vi "FieldScouting.vi"() -> ()   [LabVIEW 2015]
uses:
  <vilib>/Utility/sysdir.llb/System Directory Type.ctl
panel:
  in  "Comments":string
  in  "Low Goals Auto":dbl format="%#_4g"
  in  "High Goals Auto":dbl format="%#_4g"
  in  "?":bool
  in  "Rating":dbl=1.0 min=1.0 max=10.0 step=1.0
  in  "Low Goals":dbl format="%#_4g"
  in  "High Goals":dbl format="%#_4g"
  in  "Team Number":dbl format="%#_4g"
  in  "Scale?":bool
  in  "Auto?":bool
  in  "Tele Pass 5":bool
  in  "Tele Pass 4":bool
  in  "Tele Pass 3":bool
  in  "Tele Pass 2":bool
  in  "Tele Pass 1":bool
  in  "Auto Def 4":bool
  in  "Auto Def 3":bool
  in  "Auto Def 2":bool
  in  "Auto Def 1":bool
  in  "Touch 1":bool
  in  "Pass 5":bool
  in  "Pass 4":bool
  in  "Pass 3":bool
  in  "Pass 2":bool
  in  "Pass 1":bool
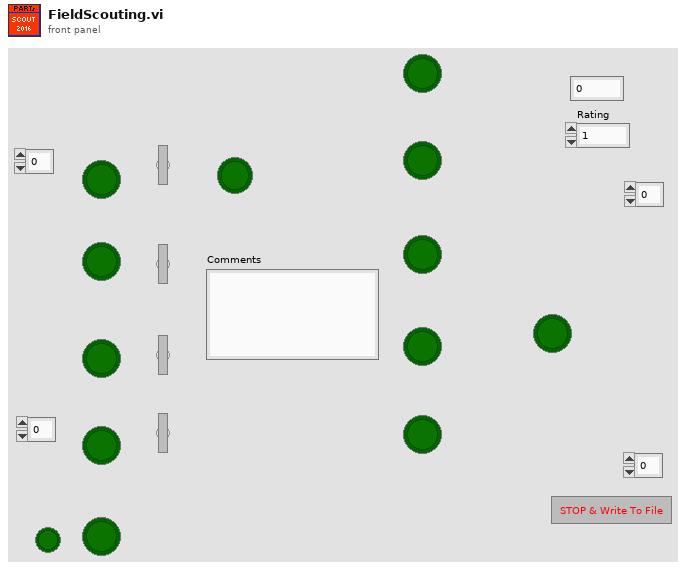
[diagram p1: front panel]
types:
  T1 = typedef "System Directory Type.ctl" = i32
  T2 = enum16{"open", "replace", "create", "open or create", "replace or create", "replace or create with confirmation"}
  T3 = enum32{"invalid app kind", "Development System", "Run Time System", "Student Edition", "Embedded LabVIEW", "Evaluation", "Custom"}
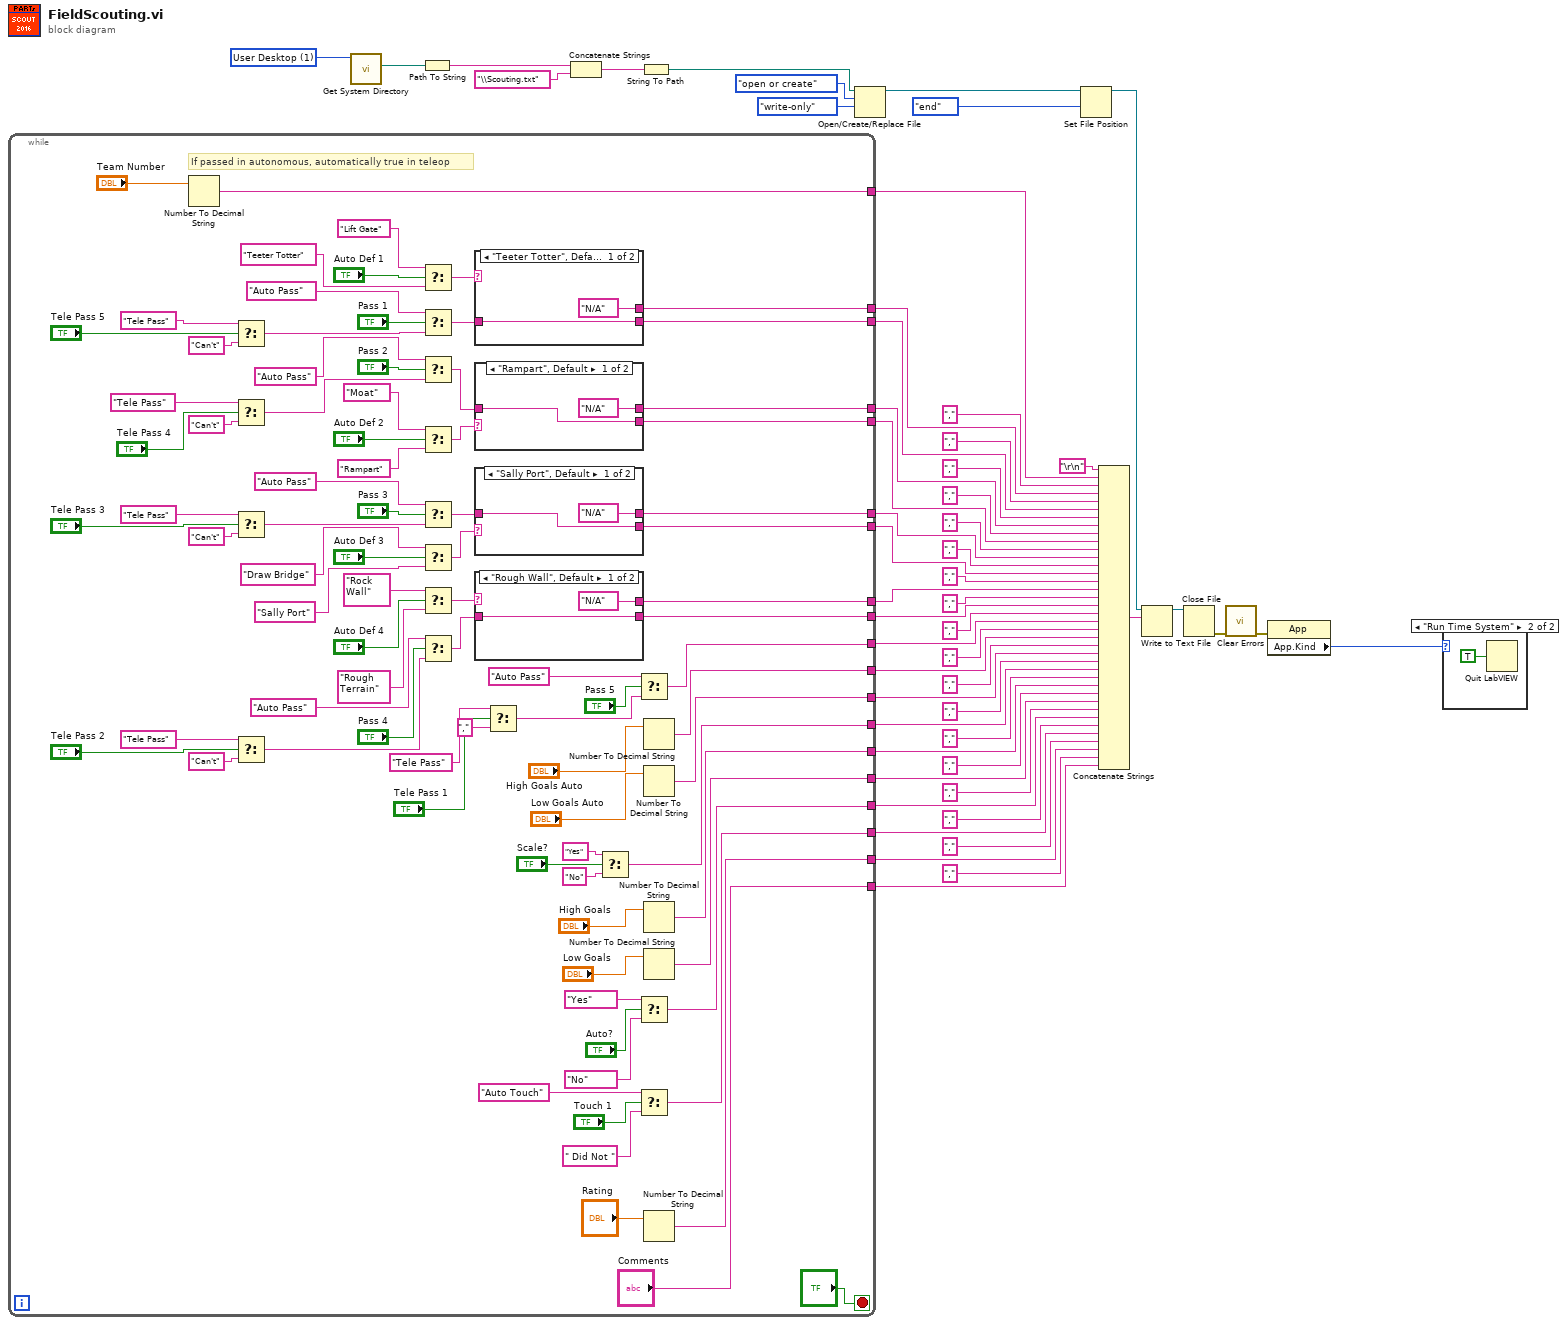
[diagram p0: block diagram]
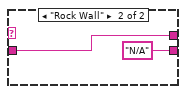
[diagram p2: hidden frame]
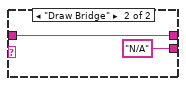
[diagram p3: hidden frame]
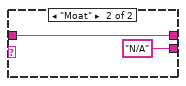
[diagram p4: hidden frame]
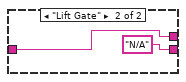
[diagram p5: hidden frame]
diagram:
  w16 = T1 1 items=["User Home"=0, "User Desktop"=1, "User Documents"=2, "User Application Data"=3, "User Preferences"=4, "User Temporary"=5, "Public Documents"=6, "Public Application Data"=7, "Public Preferences"=8, "Public Cache"=13, "System Core Libraries"=9, "System Installed Libraries"=10, "Application Files"=11, "Boot Volume Root"=12] ("system directory type")
  n1 = while {
    tunnel: [w81] -> w41
    tunnel: [w80] -> w40
    tunnel: [w79] -> w39
    tunnel: [w78] -> w38
    tunnel: [w77] -> w37
    tunnel: [w76] -> w36
    tunnel: [w75] -> w35
    tunnel: [w74] -> w34
    tunnel: [w73] -> w33
    tunnel: [w72] -> w32
    tunnel: [w58] -> w31
    tunnel: [w56] -> w27
    tunnel: [w71] -> w26
    tunnel: [w70] -> w25
    tunnel: [w69] -> w24
    tunnel: [w68] -> w23
    tunnel: [w66] -> w4
    tunnel: [w60] -> w6
    tunnel: ["Comments"] -> w1
    stop <- "?" stop-if-true
    # "If passed in autonomous, automatically true in teleop"
    n2 = Number To Decimal String(number="Team Number") -> (decimal integer string=w81:string)  [unwired: 1 in]
    n3 = Select(t="Tele Pass", s="Tele Pass 5", f="Can't") -> (s? t:f=w95:string)
    n4 = Select(t="Tele Pass", s="Tele Pass 4", f="Can't") -> (s? t:f=w93:string)
    n5 = Select(t="Tele Pass", s="Tele Pass 3", f="Can't") -> (s? t:f=w89:string)
    n6 = Select(t="Tele Pass", s="Tele Pass 2", f="Can't") -> (s? t:f=w86:string)
    n7 = Select(t="Lift Gate", s="Auto Def 1", f="Teeter Totter") -> (s? t:f=w103:string)
    n8 = Select(t="Auto Pass", s="Pass 1", f=w95) -> (s? t:f=w94:string)
    n9 = Select(t="Auto Pass", s="Pass 2", f=w93) -> (s? t:f=w92:string)
    n10 = Select(t="Moat", s="Auto Def 2", f="Rampart") -> (s? t:f=w91:string)
    n11 = Select(t="Auto Pass", s="Pass 3", f=w89) -> (s? t:f=w87:string)
    n12 = Select(t="Draw Bridge", s="Auto Def 3", f="Sally Port") -> (s? t:f=w88:string)
    n13 = Select(t="Rock Wall", s="Auto Def 4", f="Rough Terrain") -> (s? t:f=w84:string)
    n14 = Select(t="Auto Pass", s="Pass 4", f=w86) -> (s? t:f=w85:string)
    n15 = case shown="\"Teeter Totter\", Default" w103 {
      tunnel: [w153 "N/A" ("t")] -> w79
      tunnel: w94 -> [w153 w155]
      tunnel: ["N/A" w155] -> w80
      frame "Teeter Totter", Default {
      }
      frame "Lift Gate" {
      }
    }
    n16 = case shown="\"Rampart\", Default" w91 {
      tunnel: [w149 "N/A" ("t")] -> w77
      tunnel: w92 -> [w149 w151]
      tunnel: ["N/A" w151] -> w78
      frame "Rampart", Default {
      }
      frame "Moat" {
      }
    }
    n17 = case shown="\"Sally Port\", Default" w88 {
      tunnel: [w145 "N/A" ("t")] -> w75
      tunnel: w87 -> [w145 w147]
      tunnel: ["N/A" w147] -> w76
      frame "Sally Port", Default {
      }
      frame "Draw Bridge" {
      }
    }
    n18 = case shown="\"Rough Wall\", Default" w84 {
      tunnel: [w141 "N/A" ("t")] -> w73
      tunnel: w85 -> [w141 w143]
      tunnel: ["N/A" w143] -> w74
      frame "Rough Wall", Default {
      }
      frame "Rock Wall" {
      }
    }
    n19 = Select(t="Tele Pass", s="Tele Pass 1", f=",") -> (s? t:f=w82:string)
    n20 = Select(t="Yes", s="Scale?", f="No") -> (s? t:f=w71:string)
    n21 = Select(t="Auto Pass", s="Pass 5", f=w82) -> (s? t:f=w72:string)
    n22 = Select(t="Yes", s="Auto?", f="No") -> (s? t:f=w68:string)
    n23 = Select(t="Auto Touch", s="Touch 1", f=" Did Not ") -> (s? t:f=w60:string)
    n24 = Number To Decimal String(number="High Goals Auto") -> (decimal integer string=w58:string)  [unwired: 1 in]
    n25 = Number To Decimal String(number="Low Goals Auto") -> (decimal integer string=w56:string)  [unwired: 1 in]
    n26 = Number To Decimal String(number="High Goals") -> (decimal integer string=w70:string)  [unwired: 1 in]
    n27 = Number To Decimal String(number="Low Goals") -> (decimal integer string=w69:string)  [unwired: 1 in]
    n28 = Number To Decimal String(number="Rating") -> (decimal integer string=w66:string)  [unwired: 1 in]
  }
  n29 = call <vilib>:"Get System Directory.vi"("system directory type"=w16) -> ("system directory"=w15:path)  [unwired: 10 in]
  n30 = Path To String(path=w15) -> (string=w14:string)
  n31 = Concatenate Strings(w14, "\\Scouting.txt" ("string")) -> (w12:string)
  n32 = String To Path(string=w12) -> (path=w11:path)
  n33 = Open/Create/Replace File(file path (use dialog)=w11, operation (0:open)=T2."open or create", access (0:read/write)=enum16{"read/write", "read-only", "write-only"}."write-only") -> (refnum out=w19:refnum<file>)  [unwired: 3 in, 2 out]
  n34 = Set File Position(refnum=w19, from (0:start)=enum16{"start", "end", "current"}."end") -> (refnum out=w18:refnum<file>)  [unwired: 2 in, 1 out]
  n35 = Concatenate Strings("\r\n", w41, "," ("string"), w40, "," ("string"), w39, "," ("string"), w38, "," ("string"), w37, "," ("string"), w36, "," ("string"), w35, "," ("string"), w34, "," ("string"), w33, "," ("string"), w32, "," ("string"), w31, "," ("string"), w27, "," ("string"), w26, "," ("string"), w25, "," ("string"), w24, "," ("string"), w23, "," ("string"), w6, "," ("string"), w4, "," ("string"), w1) -> (w7:string)
  n36 = Write to Text File(file (use dialog)=w18, text=w7) -> (refnum out=w20:refnum<file>)  [unwired: 2 in, 2 out]
  n37 = Close File(refnum=w20) -> (error out=w10:errorcluster)  [unwired: 1 in, 1 out]
  n38 = call <vilib>:"Clear Errors.vi"("error in (no error)"=w10) -> ("error out"=w9:errorcluster)  [unwired: 5 in, 1 out]
  n39 = property class="App"(error in=w9) -> ("App.Kind"=w8:T3)  [unwired: 1 in, 2 out]
  n40 = case shown="\"Run Time System\"" w8 {
    frame Default {
    }
    frame "Run Time System" {
      n41 = Quit LabVIEW(quit? (T)=TRUE) -> ()
    }
  }
